vi "ReactorSIM.vi"(3 "Halt?":bool) -> ()   [LabVIEW 2018]
uses:
  <vilib>/Simulation/Scripting/Companion Diagram/SimConfigNode/SimParams.ctl
  <vilib>/Simulation/Scripting/Companion Diagram/SimConfigNode/_simSolvers.ctl
  <vilib>/Simulation/Implementation/Shared/SIMSCR Execution Mode.ctl
  <vilib>/Platform/TimedLoop/XDataNode/timing_clust.ctl
  <vilib>/Platform/TimedLoop/XDataNode/nitl_modes.ctl
  <vilib>/Platform/TimedLoop/XDataNode/wakeup.ctl
  <vilib>/Simulation/Param Hierarchy/Typedefs/SIMPH Param Control Actions.ctl
  <vilib>/Simulation/Implementation/Shared/SIM limit type.ctl
  <vilib>/Simulation/Scripting/Editor Utilities/SIM subVI tag data.ctl
  <vilib>/Simulation/Scripting/Editor Utilities/SIM subVI execution type.ctl
  <vilib>/Simulation/Implementation/Shared/NILVSim_ParamChanged.vi
  <vilib>/Simulation/Implementation/Shared/NILVSim_FinishedLate.vi
  <vilib>/Simulation/Implementation/Shared/NILVSIM_BeginStep.vi
  <vilib>/Simulation/Utility/Implementation/SIM Halt.vi
  <vilib>/Simulation/Utility/Implementation/SIM Time.vi
  <vilib>/Simulation/ContinuousLinear/Implementation/NILVSim Integrator new.llb/SIM Integrator distributor (scalar).vi
  <vilib>/Simulation/Implementation/Shared/SIM Fire Discrete SubVI.vi
  <vilib>/Simulation/ContinuousLinear/Implementation/NILVSim Integrator new.llb/SIM Integrator collector (scalar).vi
  <vilib>/Simulation/Implementation/Shared/NILVSim_Manager.vi
  <vilib>/Utility/error.llb/Clear Errors.vi
  <vilib>/Simulation/Implementation/Shared/NILVSim_FinalizeModel.vi
  <vilib>/Simulation/Implementation/Shared/SIM Fire Discrete SubVI (Core).vi
  <vilib>/Simulation/Implementation/Shared/SIM Unbundle Sim Info.vi
  <vilib>/Simulation/Implementation/Shared/SIMSH Read Queue.vi
  <vilib>/Simulation/Implementation/Shared/NILVSim_Initialize.vi
  <vilib>/imath/engines/lvmath2/RunTimeEngine/Managers/WorkSpace/UID Generator.vi
  <vilib>/imath/engines/lvmath2/RunTimeEngine/RunTimeType/NIMS_RunTimeType_From StrictType (excl LVString).vi
  <instcachedir>/0/NIMS_RunTimeType_From StrictType (excl LVString)_E7E34A65C99947108168652BAD14964D.lvgen/NIMS_RunTimeType_From StrictType (excl LVString)_E7E34A65C99947108168652BAD14964D_000.vi
  <vilib>/imath/engines/lvmath2/RunTimeEngine/LocalVariableDefStatement/MC_LocalVariableDefStatement_Display.vi
  <vilib>/imath/engines/lvmath2/RunTimeEngine/Managers/SymbolTable/Clear UID.vi
  <vilib>/imath/engines/lvmath2/RunTimeEngine/NodeEndStatement/NIMS_NodeEndStatement_Output.vi
  <instcachedir>/0/NIMS_NodeEndStatement_Output_53EC0D466D134D7ABD903AC30B43404B.lvgen/NIMS_NodeEndStatement_Output_53EC0D466D134D7ABD903AC30B43404B_001.vi
  <vilib>/imath/engines/lvmath2/RunTimeEngine/ErrorHandling/NIMS_Finalize Error.vi
  <instcachedir>/0/NIMS_NodeEndStatement_Output_53EC0D466D134D7ABD903AC30B43404B.lvgen/NIMS_NodeEndStatement_Output_53EC0D466D134D7ABD903AC30B43404B_009.vi
  <vilib>/Simulation/Utility/Implementation/NILVSim Get Time and IsAcceptedStep.vi
  <vilib>/Simulation/Implementation/Shared/NILVSim_GetModelError.vi
  <vilib>/Simulation/Implementation/Shared/SIM Bundle Sim Info.vi
  <vilib>/Simulation/Scripting/Companion Diagram/SimConfigNode/SimDog.xnode
  <vilib>/Platform/TimedLoop/XDataNode/XDataNode.xnode
  <vilib>/Simulation/Implementation/XNodeFramework/SimXNode/SimX.xnode
  <vilib>/Simulation/ContinuousLinear/Implementation/NILVSim Integrator new.llb/SIM Integrator (scalar).vi
  <vilib>/imath/engines/lvmath2/RunTimeEngine/Managers/SymbolTable/NIMS_WorkSpace.lvlib
  <vilib>/Platform/TimedLoop/XDataNode/XDNodeRunTimeDep.lvlib
  <vilib>/Simulation/Implementation/Shared/NI_SIM_Implementation.lvlib
panel:
  out "FJ":dbl
  out "F0":dbl
  out "F":cdb
  out "SIM-BPCS-TX-ARRAY":dbl[](array[numeric])
  out "SIM-SIS-TX-ARRAY":dbl[](array[numeric])
  out "SIM-BPCS-RX-ARRAY":dbl[](array[numeric])
  out "SIS-SIM-RX-ARRAY":bool[](array[boolean])
  out "Cooling Water Temperature":dbl(graph) caption="Reactor Level"
  out "Reactor Temperature":dbl(graph) caption="Reactor Level"
  out "Reactor Concentration":dbl(graph) caption="Reactor Level"
  out "Reactor Level":dbl(graph)
  in  "SIM Parameters":T1={"Step Size (s)"=0.01, "Final Time (s)"=700.0, "ODE Solver"=enum."Runge-Kutta 23 (variable)"}
  in  "Valve CV":cluster{"Cv":dbl, "Cv0":dbl, "CvJ":dbl}={"Cv"=4.0, "Cv0"=4.0, "CvJ"=12.336}
  in  "Reactor Disturbances":cluster{"T0":dbl, "CA0":dbl, "TJ0":dbl}={"T0"=350.0, "CA0"=1250.0, "TJ0"=300.0}
  in  "Reactor Parameters":T2={"E_R"=8330.1, "A"=1.3, "Lam"=130000.0, "Alpha"=10000000000.0, "rho"=1000000.0, "rhoj"=1000000.0, "Cp"=1.0, "CJ"=1.0, "U_AH"=2000000.0, "VJ"=10.0} {"U_AH" format="%#_6e"; "rhoj" format="%#_6e"; "rho" format="%#_6e"; "Alpha" format="%#_6e"; "Lam" format="%#_6e"}
  out "simulation time":dbl=5.2700000000000005
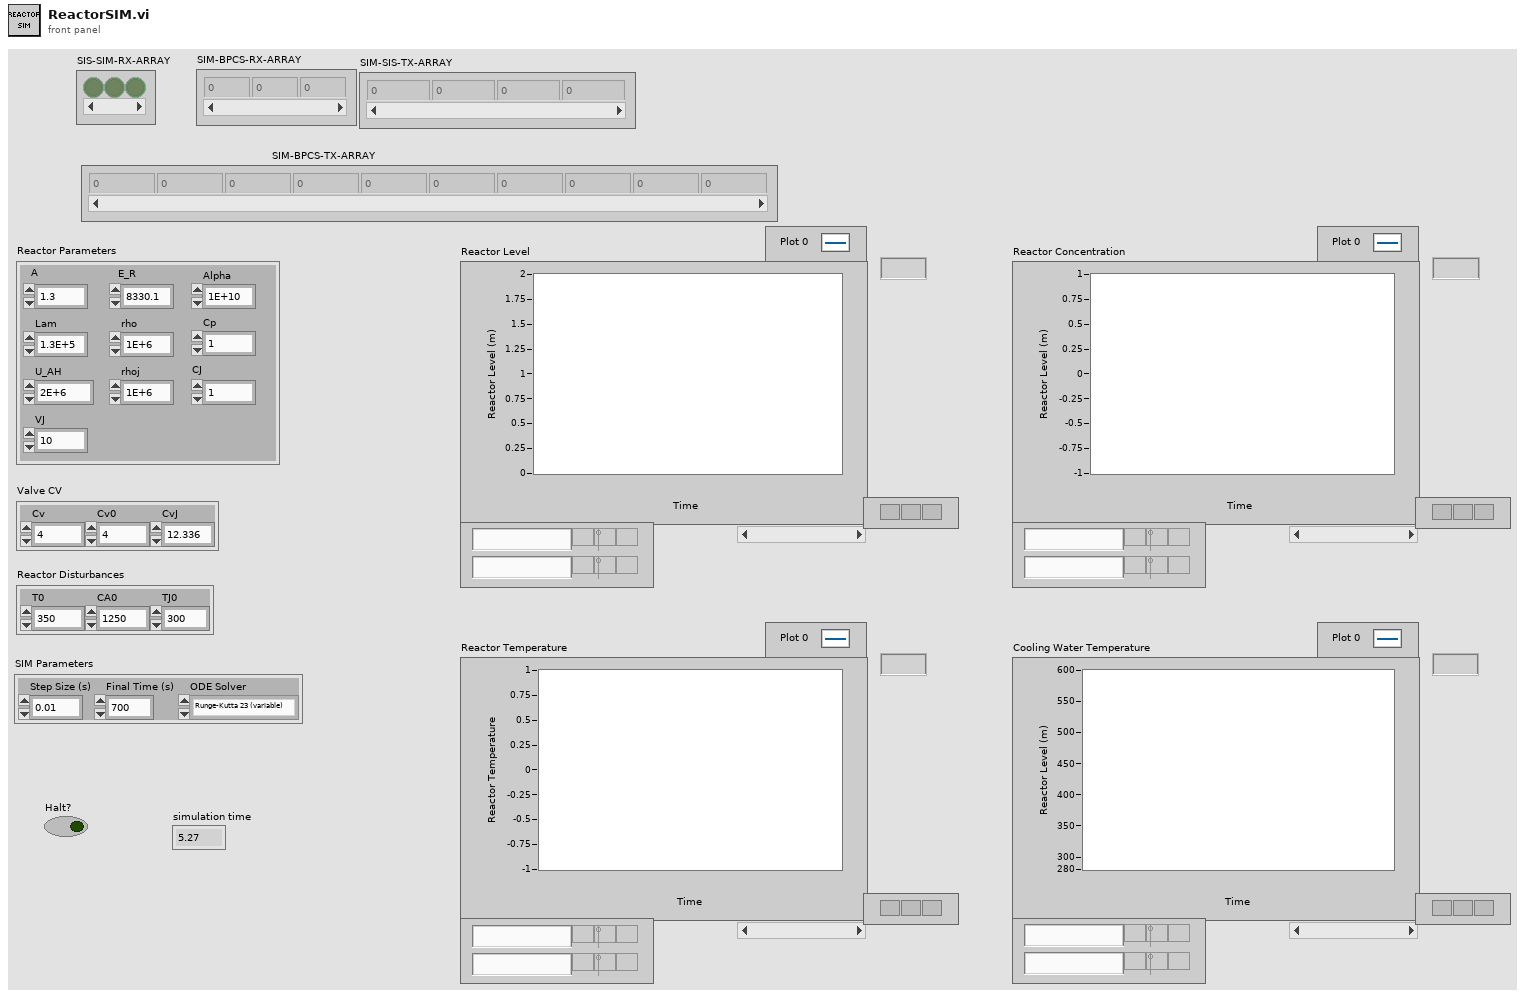
[diagram p1: front panel]
types:
  T1 = cluster{"Step Size (s)":dbl, "Final Time (s)":dbl, "ODE Solver":enum16{"Runge-Kutta 1 (Euler)", "Runge-Kutta 2", "Runge-Kutta 3", "Runge-Kutta 4", "Runge-Kutta 23 (variable)", "Runge-Kutta 45 (variable)", "BDF (variable)", "Adams-Moulton (variable)", "Rosenbrock (variable)", "Discrete States Only", "SDIRK 4 (variable)", "Radau 5 (variable)", "Radau 9 (variable)", "Radau 13 (variable)", "Radau [Variable Order] (variable)", "Gear's Method (variable)"}}
  T2 = cluster{"E_R":dbl, "A":dbl, "Lam":dbl, "Alpha":dbl, "rho":dbl, "rhoj":dbl, "Cp":dbl, "CJ":dbl, "U_AH":dbl, "VJ":dbl}
  T3 = typedef "SIMSCR Execution Mode.ctl" = enum16{"Simulate to Completion", "Single Time-Step Simulation (Fixed Step Only)"}
  T4 = typedef "XDNodeRunTimeDep.lvlib/timing_clust.ctl" = cluster{"Expected End [f-1]":u64, "Actual End [f-1]":u64, "Finished Late? [f-1]":bool, "Expected End [i-1]":u64, "Actual End [i-1]":u64, "Finished Late? [i-1]":bool, "Expected Start [i]":u64, "Actual Start [i]":u64, "Expected Start [f]":u64, "Actual Start [f]":u64, "Source Name":string, "Structure Name":string, "Period":i64, "Deadline":i64, "Offset":i64, "Start":i64, "Priority":i32, "Timeout":i32, "Mode":T5, "Wakeup Reason":T6, "Error":errorcluster, "Source Type":string, "Secondary Source Type":string, "Global End Time":u64, "Global Start Time":u64, "Frame Duration":u64, "Iteration Duration":u64, "Assigned CPU":i32, "I/O Scan Engine Mode":u32}
  T5 = typedef "XDNodeRunTimeDep.lvlib/nitl_modes.ctl" = enum32{"No Change", "Process missed periods, maintain original phase", "Discard missed periods, maintain original phase", "Process missed periods, ignore original phase", "Discard missed periods, ignore original phase"}
  T6 = typedef "XDNodeRunTimeDep.lvlib/wakeup.ctl" = enum32{"Normal", "Aborted", "Asynchronous wakeup", "Timing source error", "Timed loop error", "Timeout"}
  T7 = typedef "SIMPH Param Control Actions.ctl" = enum16{"get params", "set params"}
  T8 = typedef "SIM subVI tag data.ctl" = cluster{"period":dbl, "skew":dbl, "Simulation execution type":T9}
  T9 = typedef "SIM subVI execution type.ctl" = enum16{"Function call", "Discrete", "Continuous", "Initialization only", "Final step only"}
  T10 = typedef "SIM limit type.ctl" = enum16{"upper", "lower", "both", "none"}
  T11 = typedef "SimParams.ctl" = cluster{"Initial Time (s)":dbl, "Final Time (s)":dbl, "Step Size (s)":dbl, "ODE Solver":T12, "Minimum Step Size (s)":dbl, "Maximum Step Size (s)":dbl, "Relative Tolerance":dbl, "Absolute Tolerance":dbl, "Software Timing":bool, "Initial Step Size (s)":dbl, "Automatic Fixed Step Size?":bool, "Automatic Discrete Step Size?":bool, "Discrete Step Size (s)":dbl, "Calculate using Time Step":bool, "Solver Wired?":bool, "Prev.Frm.Expected End":u64, "Prev.Frm.Actual End":u64, "Prev.Frm.Finished Late?":bool, "Prev.Iter.Expected End":u64, "Prev.Iter.Actual End":u64, "Prev.Iter.Finished Late?":bool, "Expected Iteration Start":u64, "Actual Iteration Start":u64, "Expected Frame Start":u64, "Actual Frame Start":u64, "Source Name":string, "Name":string, "Period":i64, "Deadline":i64, "Offset":i64, "Start":i64, "Priority":i32, "Timeout":i32, "Processor":i32, "Mode":enum32{"No Change", "Process missed periods, maintain original phase", "Discard missed periods, maintain original phase", "Process missed periods, ignore original phase", "Discard missed periods, ignore original phase"}, "Wakeup reason":enum32{"Normal", "Aborted", "Asynchronous wakeup", "Timing source error", "Timed loop error", "Timeout"}, "Error":errorcluster, "Source Type":string, "Secondary Source Type":string, "Global End Time":u64, "Global Start Time":u64, "Full Solver Reset":bool, "Execution Mode":T3, "Nan/Inf Check":bool, "Custom Solver Library":string, "Solver Is Variable":bool, "custom solver name":string, "Signal Collection Decimation":u32}
  T12 = typedef "_simSolvers.ctl" = enum16{"Runge-Kutta 1 (Euler)", "Runge-Kutta 2", "Runge-Kutta 3", "Runge-Kutta 4", "Runge-Kutta 23 (variable)", "Runge-Kutta 45 (variable)", "BDF (variable)", "Adams-Moulton (variable)", "Rosenbrock (variable)", "Discrete States Only", "SDIRK 4 (variable)", "Radau 5 (variable)", "Radau 9 (variable)", "Radau 13 (variable)", "Radau [Variable Order] (variable)", "Gear's Method (variable)", "Linearizer", "State Query", "Trim Eval", "Custom Solver"}
  T13 = enum16{"Runge-Kutta 1 (Euler)", "Runge-Kutta 2", "Runge-Kutta 3", "Runge-Kutta 4", "Runge-Kutta 23 (variable)", "Runge-Kutta 45 (variable)", "BDF (variable)", "Adams-Moulton (variable)", "Rosenbrock (variable)", "Discrete States Only", "SDIRK 4 (variable)", "Radau 5 (variable)", "Radau 9 (variable)", "Radau 13 (variable)", "Radau [Variable Order] (variable)", "Gear's Method (variable)"}
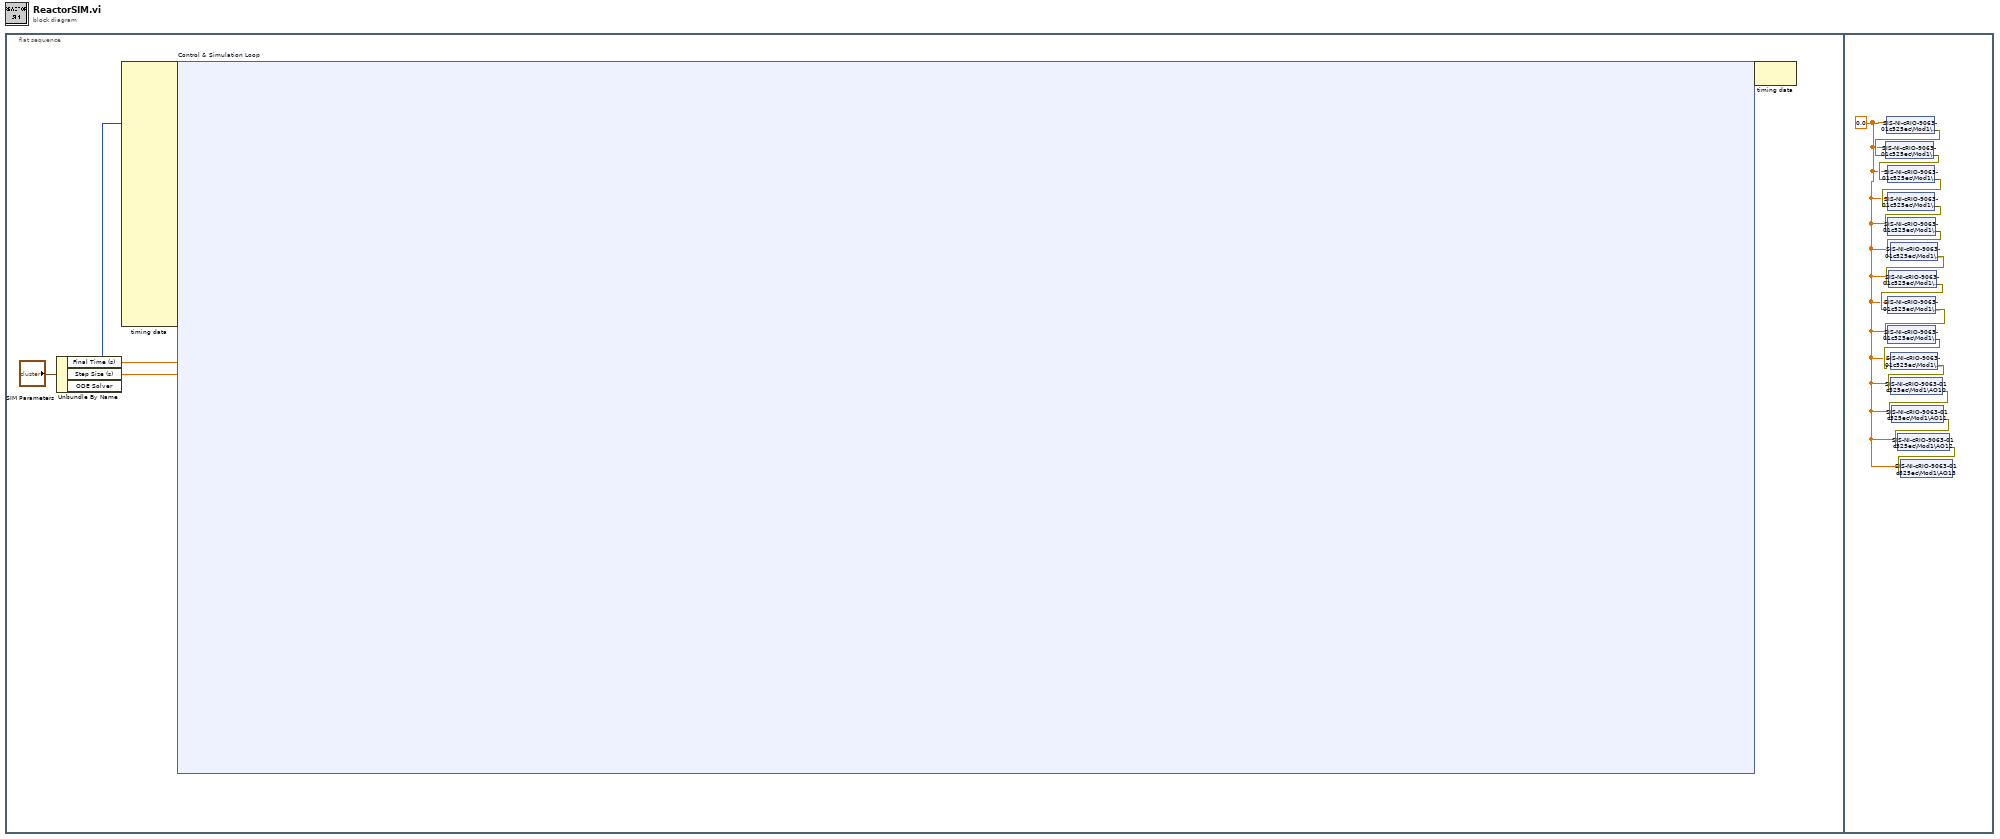
[diagram p0: block diagram]
diagram:
  n1 = flat-sequence {
    frame #0 {
      n2 = Unbundle By Name ("Unbundle By Name 3")("SIM Parameters") -> ("Final Time (s)"=w1:dbl, "Step Size (s)"=w2:dbl, "ODE Solver"=w3:T13)
      n3 = node-c288(w1, w2, w3) -> (w6:variant)  [unwired: 21 in]
      n4 = node-c254 "Control & Simulation Loop"(w6) -> (w5:variant)
      n5 = node-c288(w5) -> ()  [unwired: 1 out]
    }
    frame #1 {
      w1779 = 0.0 ("AO0")
      n6 = shared-variable "SIS-NI-cRIO-9063-01c525ec\\Mod1\\AO0"(w1779) -> (error out=w1792:errorcluster)  [unwired: 1 in]
      n7 = shared-variable "SIS-NI-cRIO-9063-01c525ec\\Mod1\\AO1"(w1779, error in=w1792) -> (error out=w1791:errorcluster)
      n8 = shared-variable "SIS-NI-cRIO-9063-01c525ec\\Mod1\\AO2"(w1779, error in=w1791) -> (error out=w1790:errorcluster)
      n9 = shared-variable "SIS-NI-cRIO-9063-01c525ec\\Mod1\\AO3"(w1779, error in=w1790) -> (error out=w1789:errorcluster)
      n10 = shared-variable "SIS-NI-cRIO-9063-01c525ec\\Mod1\\AO4"(w1779, error in=w1789) -> (error out=w1788:errorcluster)
      n11 = shared-variable "SIS-NI-cRIO-9063-01c525ec\\Mod1\\AO5"(w1779, error in=w1788) -> (error out=w1787:errorcluster)
      n12 = shared-variable "SIS-NI-cRIO-9063-01c525ec\\Mod1\\AO6"(w1779, error in=w1787) -> (error out=w1786:errorcluster)
      n13 = shared-variable "SIS-NI-cRIO-9063-01c525ec\\Mod1\\AO7"(w1779, error in=w1786) -> (error out=w1785:errorcluster)
      n14 = shared-variable "SIS-NI-cRIO-9063-01c525ec\\Mod1\\AO8"(w1779, error in=w1785) -> (error out=w1784:errorcluster)
      n15 = shared-variable "SIS-NI-cRIO-9063-01c525ec\\Mod1\\AO9"(w1779, error in=w1784) -> (error out=w1783:errorcluster)
      n16 = shared-variable "SIS-NI-cRIO-9063-01c525ec\\Mod1\\AO10"(w1779, error in=w1783) -> (error out=w1782:errorcluster)
      n17 = shared-variable "SIS-NI-cRIO-9063-01c525ec\\Mod1\\AO11"(w1779, error in=w1782) -> (error out=w1781:errorcluster)
      n18 = shared-variable "SIS-NI-cRIO-9063-01c525ec\\Mod1\\AO12"(w1779, error in=w1781) -> (error out=w1780:errorcluster)
      n19 = shared-variable "SIS-NI-cRIO-9063-01c525ec\\Mod1\\AO13"(w1779, error in=w1780) -> ()  [unwired: 1 out]
    }
  }
